vi "Tray_BtnArrCreate.vi"(8 "error in":errorcluster, 9 "MaxArea":cluster{"x":u32, "y":u32}={"x"=10, "y"=10}, 10 "GridSize":cluster{"x":u32, "y":u32}={"x"=10, "y"=10}, 11 "Refin":T1) -> (0 "error out":errorcluster)   [LabVIEW 2019]
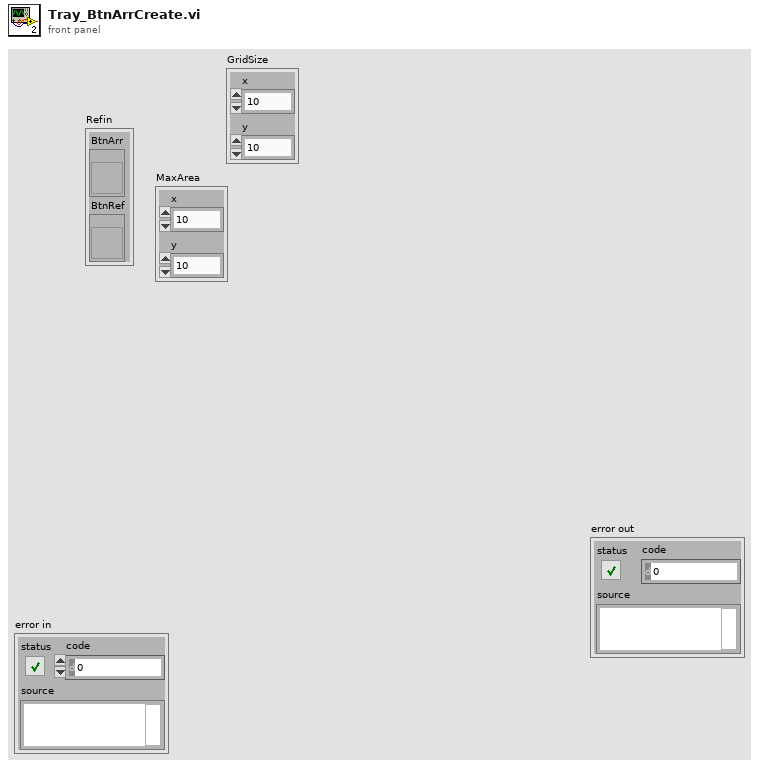
[diagram p1: front panel]
types:
  T1 = cluster{"BtnArr":refnum<vi>, "BtnRef":refnum<vi>}
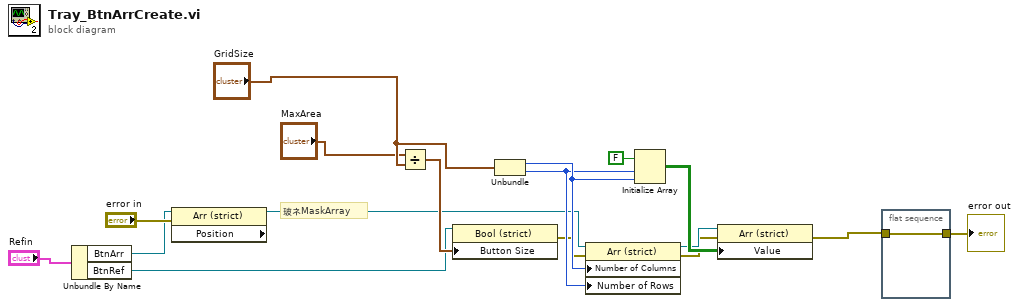
[diagram p0: block diagram]
diagram:
  # "玻ネMaskArray"
  n1 = Unbundle By Name("Refin") -> ("BtnArr"=w1:refnum<vi>, "BtnRef"=w11:refnum<vi>)
  n2 = property on="Property Node" class="Arr (strict)" props=["Position"](reference=w1, error in="error in") -> (reference out=w8:refnum<vi>)  [unwired: 2 out]
  n3 = Divide(x="MaxArea", y="GridSize") -> (x/y=w12:cluster{"x":dbl, "y":dbl})
  n4 = property on="Property Node" class="Bool (strict)"(reference=w11, "Button Size"=w12) -> (error out=w13:errorcluster)  [unwired: 1 in, 1 out]
  n5 = Unbundle("GridSize") -> ("x"=w17:u32, "y"=w16:u32)
  n6 = property on="Property Node" class="Arr (strict)"(reference=w8, error in=w13, "Number of Columns"=w17, "Number of Rows"=w16) -> (reference out=w10:refnum<vi>, error out=w9:errorcluster)
  n7 = Initialize Array(FALSE, w16, w17) -> (w15:bool[][])
  n8 = property class="Arr (strict)"(reference=w10, error in=w9, "Value"=w15) -> (error out=w2:errorcluster)  [unwired: 1 out]
  n9 = flat-sequence {
    tunnel: w2 -> [w18]
    tunnel: [w18] -> w7
    frame #0 {
    }
  }
  "error out" <- w7
